vi "SV Average Spectra.vi"   [LabVIEW 2017]
doc: "Computes the linear RMS-averaged power spectrum of <B>scaled signal [EU]</B> in a linear scale. Use the power spectrum to quantify signal components as a function of frequency. Use this VI on embedded targets that have limited computational resources. Wire data to the <B>scaled signal [EU]</B> input to determine the polymorphic instance to use or manually select the instance."
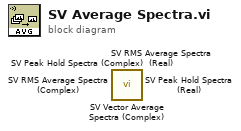
[diagram p0: block diagram]
diagram:
  n1 = call <vilib>:"SV Vector Average Spectra (Complex).vi"() -> ()  [unwired: 17 in, 3 out]
  n2 = call <vilib>:"SV RMS Average Spectra (Real).vi"() -> ()  [unwired: 15 in, 5 out]
  n3 = call <vilib>:"SV RMS Average Spectra (Complex).vi"() -> ()  [unwired: 16 in, 4 out]
  n4 = call <vilib>:"SV Peak Hold Spectra (Real).vi"() -> ()  [unwired: 15 in, 5 out]
  n5 = call <vilib>:"SV Peak Hold Spectra (Complex).vi"() -> ()  [unwired: 16 in, 4 out]
